vi "save_bin2.vi"(1 "ArrayOut":waveform(i16)[](array[waveform]), 2 "Current time":timestamp, 3 "Object":string) -> (0 "error out":errorcluster)   [LabVIEW 2010]
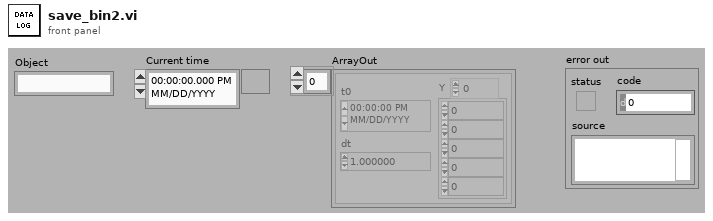
[diagram p1: front panel]
types:
  T1 = enum16{"open", "replace", "create", "open or create", "replace or create", "replace or create with confirmation"}
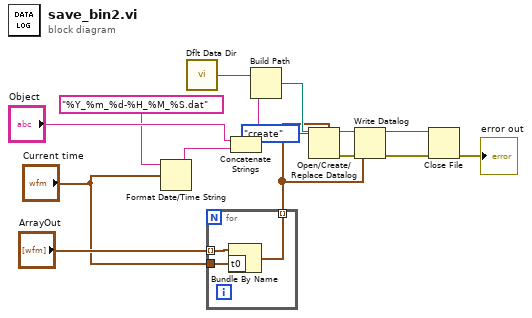
[diagram p0: block diagram]
diagram:
  n1 = Format Date/Time String(time format string (%c)="%Y_%m_%d-%H_%M_%S.dat", seconds (now)="Current time") -> (date/time string=w10:string)  [unwired: 1 in]
  n2 = call <vilib>:"Dflt Data Dir.vi"() -> ("App:Default Data Directory"=w11:path)
  n3 = for {
    tunnel: "ArrayOut" -> [w18] mode=indexing
    tunnel: "Current time" -> [w17]
    tunnel: [w16] -> w2 mode=indexing
    n4 = Bundle By Name(cluster=w18, "t0"=w17) -> (w16:waveform(i16))
  }
  n5 = Concatenate Strings("Object", w10) -> (w9:string)
  n6 = Build Path(base path=w11, name or relative path=w9) -> (appended path=w14:path)
  n7 = Open/Create/Replace Datalog(5:w2, 10:T1."create" ("operation (0:open)"), 11:w14) -> (0:w6:errorcluster, 3:w5:refnum<k1>)  [unwired: 3 in, 1 out]
  n8 = Write Datalog(4:w6, 6:w2, 7:w5) -> (0:w7:errorcluster, 3:w8:refnum<k1>)
  n9 = Close File(refnum=w8, error in=w7) -> (error out=→"error out":errorcluster)  [unwired: 1 out]
